vi "Conti CAN.vi"(8 "Error IN":errorcluster, 11 "CMD":u16) -> (0 "Error OUT":errorcluster)   [LabVIEW 2013]
uses:
  Type Defs/CAN Mode.ctl
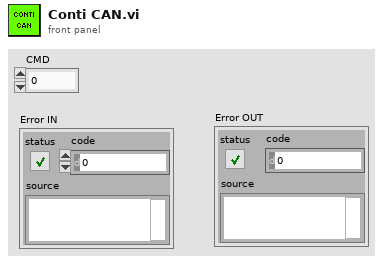
[diagram p1: front panel]
types:
  T1 = typedef "CAN Mode.ctl" = enum16{"Init", "Read", "Write", "Close"}
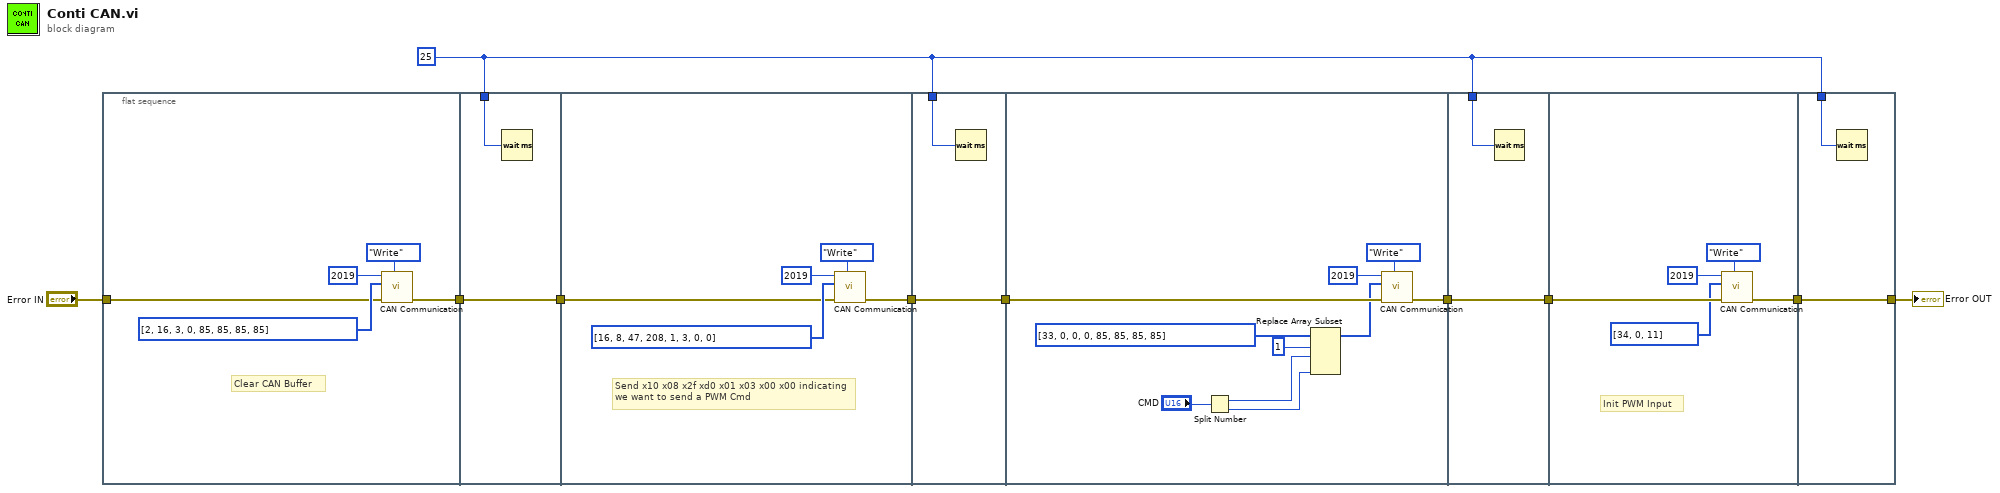
[diagram p0: block diagram]
diagram:
  w4 = u32 25 ("milliseconds to wait")
  n1 = flat-sequence {
    tunnel: [w12] -> w9
    tunnel: "Error IN" -> [w11]
    tunnel: w4 -> [w17]
    tunnel: [w16] -> w10
    tunnel: w9 -> [w16]
    tunnel: w10 -> [w19]
    tunnel: [w18] -> w7
    tunnel: w4 -> [w24]
    tunnel: [w23] -> w8
    tunnel: w7 -> [w23]
    tunnel: w8 -> [w32]
    tunnel: [w25] -> w5
    tunnel: w4 -> [w36]
    tunnel: [w35] -> w6
    tunnel: w5 -> [w35]
    tunnel: w6 -> [w39]
    tunnel: [w37] -> w3
    tunnel: w4 -> [w43]
    tunnel: [w42] -> w2
    tunnel: w3 -> [w42]
    frame #0 {
      # "Clear CAN Buffer"
      n2 = call "CAN Communication.vi"("CAN Mode"=CAN_Mode."Write", "Error IN"=w11, "Message"=u8[] [2, 16, 3, 0, 85, 85, 85, 85] ("array"), "Arbitration ID"=u32 2019 ("CAN Addres to Xmit\nSpeed CMD (Hex) 2")) -> ("Error OUT"=w12:errorcluster)  [unwired: 6 in, 1 out]
    }
    frame #1 {
      n3 = Wait (ms)(milliseconds to wait=w17) -> ()  [unwired: 1 out]
    }
    frame #2 {
      # "Send x10 x08 x2f xd0 x01 x03 x00 x00 indicating\nwe want to send a PWM Cmd"
      n4 = call "CAN Communication.vi"("CAN Mode"=CAN_Mode."Write", "Error IN"=w19, "Message"=u8[] [16, 8, 47, 208, 1, 3, 0, 0] ("array"), "Arbitration ID"=u32 2019 ("CAN Addres to Xmit\nSpeed CMD (Hex) 2")) -> ("Error OUT"=w18:errorcluster)  [unwired: 6 in, 1 out]
    }
    frame #3 {
      n5 = Wait (ms)(milliseconds to wait=w24) -> ()  [unwired: 1 out]
    }
    frame #4 {
      n6 = Split Number(x="CMD") -> (hi(x)=w28:u8, lo(x)=w27:u8)
      n7 = Replace Array Subset(array=u8[] [33, 0, 0, 0, 85, 85, 85, 85], new element #1=w28, index #1=1 ("index"), new element #2=w27) -> (w26:u8[])  [unwired: 1 in]
      n8 = call "CAN Communication.vi"("CAN Mode"=CAN_Mode."Write", "Error IN"=w32, "Message"=w26, "Arbitration ID"=u32 2019 ("CAN Addres to Xmit\nSpeed CMD (Hex) 2")) -> ("Error OUT"=w25:errorcluster)  [unwired: 6 in, 1 out]
    }
    frame #5 {
      n9 = Wait (ms)(milliseconds to wait=w36) -> ()  [unwired: 1 out]
    }
    frame #6 {
      # "Init PWM Input"
      n10 = call "CAN Communication.vi"("CAN Mode"=CAN_Mode."Write", "Error IN"=w39, "Message"=u8[] [34, 0, 11] ("array"), "Arbitration ID"=u32 2019 ("CAN Addres to Xmit\nSpeed CMD (Hex) 2")) -> ("Error OUT"=w37:errorcluster)  [unwired: 6 in, 1 out]
    }
    frame #7 {
      n11 = Wait (ms)(milliseconds to wait=w43) -> ()  [unwired: 1 out]
    }
  }
  "Error OUT" <- w2
